vi "Config Sampling Measurements - VSU name converter.vi"(1 "unit to configure":u32(slide) max=5 scale=0.0..1.0) -> (0 "VSU to be configured":string)   [LabVIEW 2016]
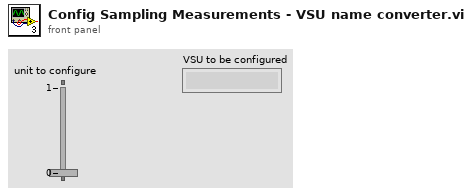
[diagram p1: front panel]
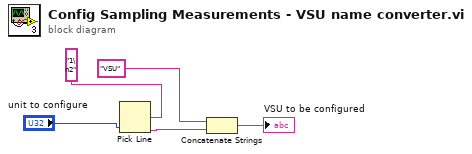
[diagram p0: block diagram]
diagram:
  n1 = Pick Line(multi-line string="1\n2", line index="unit to configure") -> (output string=w2:string)  [unwired: 1 in]
  n2 = Concatenate Strings("VSU", w2) -> (→"VSU to be configured":string)
